vi "Analysis Controller.vi"(11 "Error In":errorcluster) -> (4 "Phontation Threshold Pressure?":bool, 6 "Vocal Efficiency?":bool, 8 "Pecent Jitter and Shimmer?":bool, 10 "Phontation Threshold Flow?":bool, 15 "Error Out":errorcluster)   [LabVIEW 2015, in "SubVIs.lvlib"]
uses:
  SubVIs.lvlib
panel:
  in  "OK Go":bool
  in  "Select All":bool
  in  "Phontation Threshold Flow":bool
  in  "Phontation Threshold Pressure":bool
  in  "Pecent Jitter and Shimmer":bool
  in  "Vocal Efficiency":bool
  # "Select Desired Analysis Parameters"
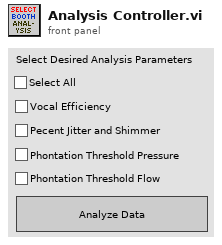
[diagram p1: front panel]
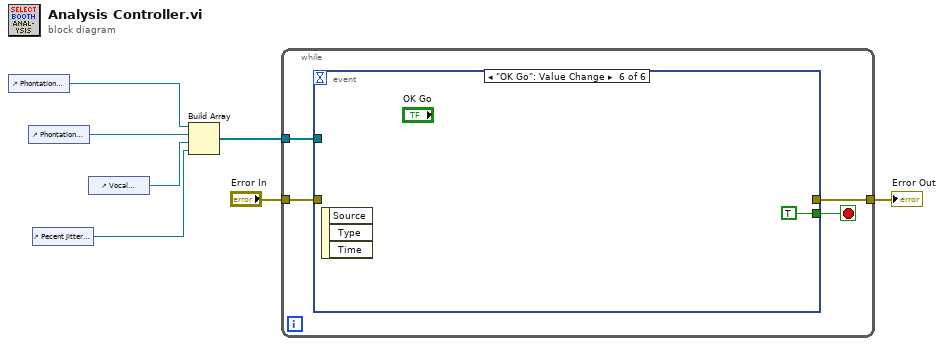
[diagram p0: block diagram]
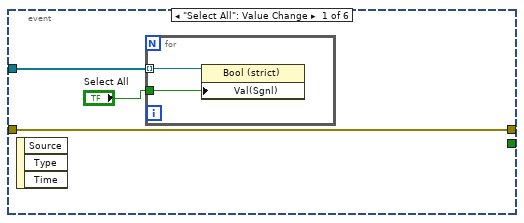
[diagram p2: hidden frame]
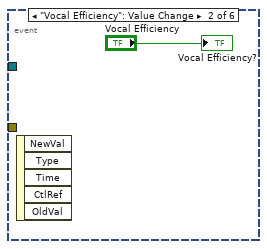
[diagram p3: hidden frame]
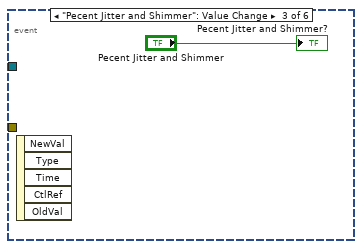
[diagram p4: hidden frame]
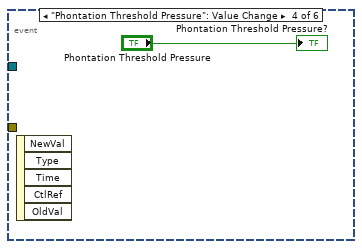
[diagram p5: hidden frame]
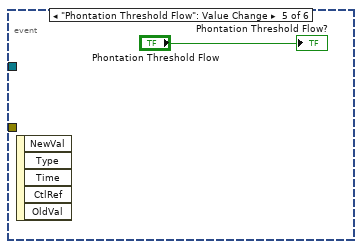
[diagram p6: hidden frame]
diagram:
  n1 = control-ref of="Phontation Threshold Pressure"() -> (w6:refnum<vi>)
  n2 = control-ref of="Phontation Threshold Flow"() -> (w5:refnum<vi>)
  n3 = control-ref of="Pecent Jitter and Shimmer"() -> (w3:refnum<vi>)
  n4 = control-ref of="Vocal Efficiency"() -> (w4:refnum<vi>)
  n5 = Build Array(w6, w5, w4, w3) -> (w7:refnum<vi>[])
  n6 = while {
    tunnel: w7 -> [w10]
    tunnel: [w9] -> w2
    tunnel: "Error In" -> [w8]
    stop <- w11 stop-if-true
    n7 = event shown="[5] \"OK Go\": Value Change" {
      selector: _ -> [_ _ _ _ _ _]
      dyn-events: _ -> [_ _ _ _ _ _]
      timeout: _ -> [_ _ _ _ _ _]
      tunnel: [_ _ _ _ _ TRUE] -> w11
      tunnel: w10 -> [w14 _ _ _ _ _]
      tunnel: [w12 _ _ _ _ _] -> w9
      tunnel: w8 -> [w12 _ _ _ _ _]
      event "Select All": Value Change {
        n8 = event-data() -> ()  [unwired: 1 in, 3 out]
        n9 = for {
          tunnel: w14 -> [w16] mode=indexing
          tunnel: "Select All" -> [w15]
          n10 = property class="Bool (strict)"(reference=w16, "Val(Sgnl)"=w15) -> ()  [unwired: 1 in, 2 out]
        }
      }
      event "Vocal Efficiency": Value Change {
        n11 = event-data() -> ()  [unwired: 1 in, 5 out]
        "Vocal Efficiency?" <- "Vocal Efficiency"
      }
      event "Pecent Jitter and Shimmer": Value Change {
        n12 = event-data() -> ()  [unwired: 1 in, 5 out]
        "Pecent Jitter and Shimmer?" <- "Pecent Jitter and Shimmer"
      }
      event "Phontation Threshold Pressure": Value Change {
        n13 = event-data() -> ()  [unwired: 1 in, 5 out]
        "Phontation Threshold Pressure?" <- "Phontation Threshold Pressure"
      }
      event "Phontation Threshold Flow": Value Change {
        n14 = event-data() -> ()  [unwired: 1 in, 5 out]
        "Phontation Threshold Flow?" <- "Phontation Threshold Flow"
      }
      event "OK Go": Value Change {
        n15 = event-data() -> ()  [unwired: 1 in, 3 out]
      }
    }
  }
  "Error Out" <- w2
